vi "intSquare.vi"(8 "Error in (no error)":errorcluster, 11 "Int in":refnum<class "IntClass.lvclass">) -> (0 "Error out":errorcluster, 1 "Timing":u32, 3 "Int out":refnum<class "IntClass.lvclass">)   [LabVIEW 2011, in "IntClass.lvclass"]
uses:
  IntClass.lvclass
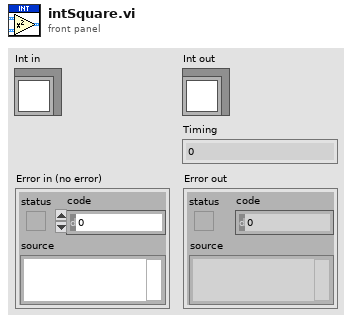
[diagram p1: front panel]
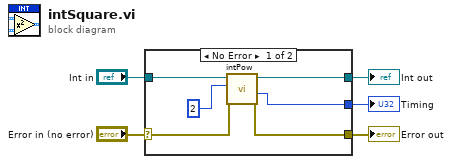
[diagram p0: block diagram]
diagram:
  n1 = case shown="No Error" "Error in (no error)" {
    selector: "Error in (no error)" -> [w9 w12]
    tunnel: "Int in" -> [w11 _]
    tunnel: [w8 w12] -> w3
    tunnel: [w10 _] -> w2
    tunnel: [w6 _] -> w1
    frame No Error {
      n2 = call "intPow.vi"("Error in (no error)"=w9, "Exponent"=u32 2, "Int in"=w11) -> ("Error out"=w8:errorcluster, "Timing"=w6:u32, "Int out"=w10:refnum<class "IntClass.lvclass">)  [unwired: 6 in]
    }
    frame Error {
    }
  }
  "Int out" <- w2
  "Error out" <- w3
  "Timing" <- w1
